vi "Extract Data From Excel.vi"(8 "error in (no error)":errorcluster, 11 "Path":path) -> (0 "error out":errorcluster, 3 "all rows":string[][](array[string]))   [LabVIEW 2021, in "User Interface.lvlib"]
uses:
  User Interface.lvlib
  <vilib>/Utility/file.llb/Read Delimited Spreadsheet (string).vi
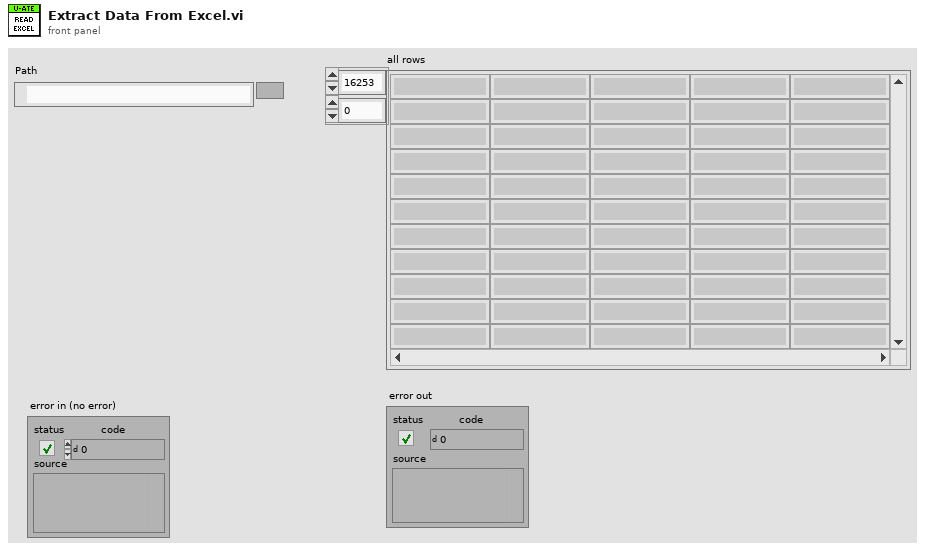
[diagram p1: front panel]
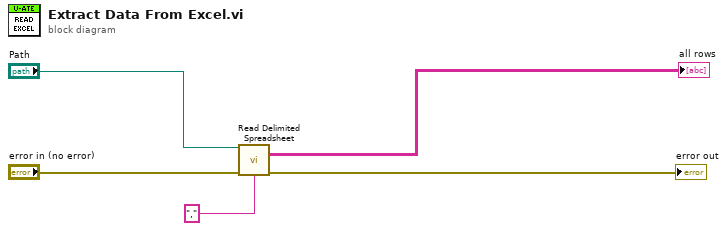
[diagram p0: block diagram]
diagram:
  n1 = call-poly <vilib>:"Read Delimited Spreadsheet.vi"("file path (dialog if empty)"="Path", "error in (no error)"="error in (no error)", "delimiter (\\t)"="," ("delimiter (\\t)")) -> ("all rows"=→"all rows":string[][], "error out"=→"error out":errorcluster)  [unwired: 7 in, 4 out]
